vi "Seconds to HHHHMMSS Strings 3.vi"(3 "mSEC":bool, 4 "hrs lead #zeros":u16, 5 "Seconds":ext format="%.2f") -> (0 "HHHHMMSS":string, 2 "HHHH:MM:SS":string)   [LabVIEW 2020]
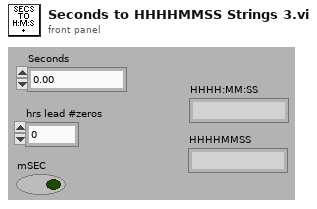
[diagram p1: front panel]
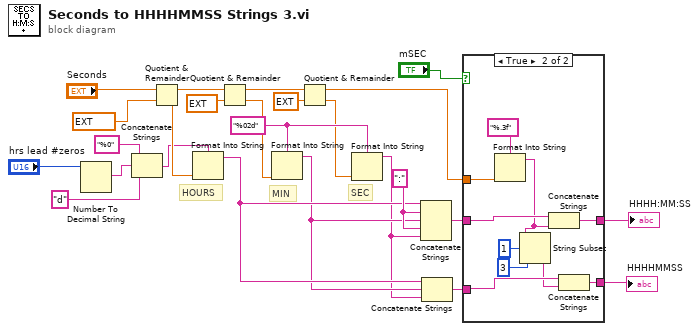
[diagram p0: block diagram]
diagram:
  w20 = "%02d" ("Format String")
  w21 = ":"
  # "SEC"
  # "MIN"
  # "HOURS"
  n1 = Number To Decimal String(number="hrs lead #zeros") -> (decimal integer string=w3:string)  [unwired: 1 out]
  n2 = Concatenate Strings("%0" ("initial string"), w3, "d" ("initial string")) -> (w1:string)
  n3 = Quotient & Remainder(x="Seconds", y=ext 3600.0) -> (x-y*floor(x/y)=w23:ext, floor(x/y)=w19:ext)
  n4 = Format Into String(format string=w1, w19) -> (resulting string=w14:string)  [unwired: 2 in, 1 out]
  n5 = Quotient & Remainder(x=w23, y=ext 60.0) -> (x-y*floor(x/y)=w22:ext, floor(x/y)=w18:ext)
  n6 = Format Into String(format string=w20, w18) -> (resulting string=w13:string)  [unwired: 2 in, 1 out]
  n7 = Quotient & Remainder(x=w22, y=ext 1.0) -> (x-y*floor(x/y)=w11:ext, floor(x/y)=w15:ext)
  n8 = Format Into String(format string=w20, w15) -> (resulting string=w12:string)  [unwired: 2 in, 1 out]
  n9 = Concatenate Strings(w14, w21, w13, w21, w12) -> (w10:string)
  n10 = Concatenate Strings(w14, w13, w12) -> (w8:string)
  n11 = case shown="True" "mSEC" {
    tunnel: w11 -> [_ w37]
    tunnel: w10 -> [w27 w35]
    tunnel: [w27 w34] -> w9
    tunnel: w8 -> [w26 w30]
    tunnel: [w26 w28] -> w7
    frame False {
    }
    frame True {
      n12 = Format Into String(format string="%.3f", w37) -> (resulting string=w33:string)  [unwired: 2 in, 1 out]
      n13 = String Subset(string=w33, offset (0)=1, length (rest)=3 ("length (rest)")) -> (substring=w29:string)
      n14 = Concatenate Strings(w35, w33) -> (w34:string)
      n15 = Concatenate Strings(w30, w29) -> (w28:string)
    }
  }
  "HHHH:MM:SS" <- w9
  "HHHHMMSS" <- w7
